vi "y_rotmatrix.vi"(1 "y-angle":dbl format="%.2f") -> (0 "y-matrix":dbl[][](array[numeric])=[[1.0, 0.0, -0.0, 0.0], [0.0, 1.0, 0.0, 0.0], [0.0, 0.0, 1.0, 0.0], [0.0, 0.0, 0.0, 1.0]] format="%.2f")   [LabVIEW 2011]
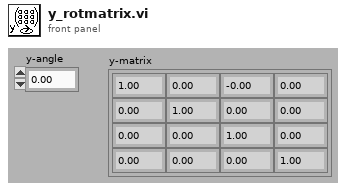
[diagram p1: front panel]
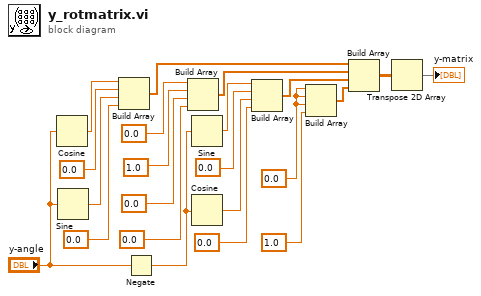
[diagram p0: block diagram]
diagram:
  w2 = 0.0
  n1 = Cosine(x="y-angle") -> (cos(x)=w15:dbl)
  n2 = Sine(x="y-angle") -> (sin(x)=w16:dbl)
  n3 = Build Array(w15, 0.0, w16, 0.0) -> (w20:dbl[])
  n4 = Negate(x="y-angle") -> (-x=w13:dbl)
  n5 = Build Array(0.0, 1.0, 0.0, 0.0) -> (w21:dbl[])
  n6 = Sine(x=w13) -> (sin(x)=w12:dbl)
  n7 = Cosine(x=w13) -> (cos(x)=w19:dbl)
  n8 = Build Array(w12, 0.0, w19, 0.0) -> (w22:dbl[])
  n9 = Build Array(w2, w2, w2, 1.0) -> (w6:dbl[])
  n10 = Build Array(w20, w21, w22, w6) -> (w8:dbl[][])
  n11 = Transpose 2D Array(2D array=w8) -> (transposed array=→"y-matrix":dbl[][])
